vi "__Test_LvDataToMemory_PTR.vi"() -> ()   [LabVIEW 2019]
uses:
  Private/LvDataToMemory_PTR.vi
  __cvi/__TEST_CVI_Prj_PTR/TEST_DataType.dll
  Memory Data Access.lvlib
panel:
  out "Ret_Cluster":i32
  out "Ret_ArrayWav":u32
  out "Ret_Waveform":u32
  out "Ret_TimeStamp":dbl
  out "Ret_ArrayStr":u32
  out "ByteArray":u8[](array[numeric])
  out "Ret_ArrayDBL":u32
  out "Ret_Path":i32
  out "Ret_Str":i32
  out "Ret_Boolean":u8
  out "Ret_DBL":dbl
  out "Ret_I32":i32
  out "Ret_U32":u32
  in  "Enum":T1(ring)
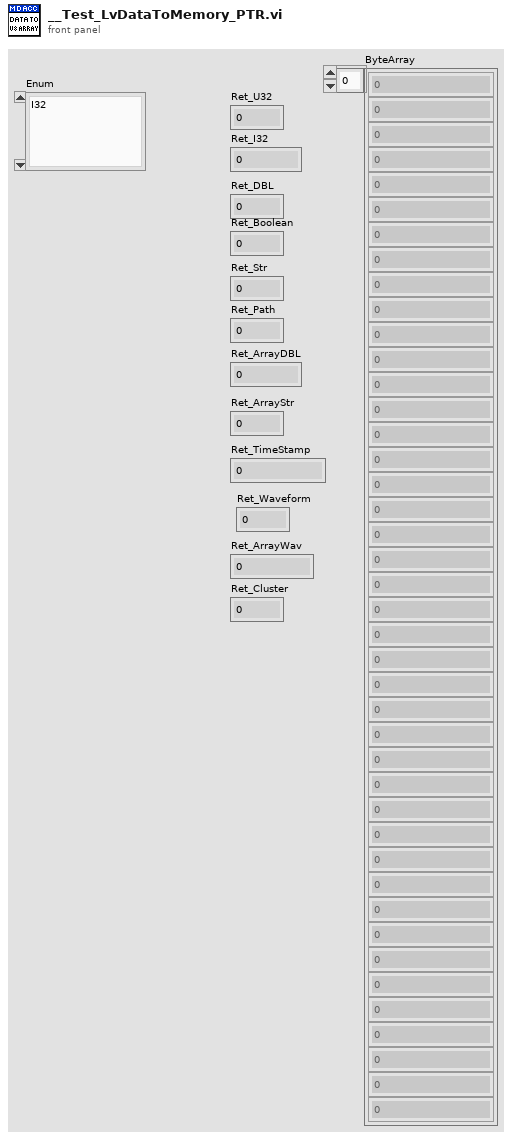
[diagram p1: front panel]
types:
  T1 = enum16{"I32", "U32", "DBL", "String", "Cluster", "Array_Str", "Array_DBL", "Array_Waveform", "Bool", "TimeStamp", "Waveform", "Path"}
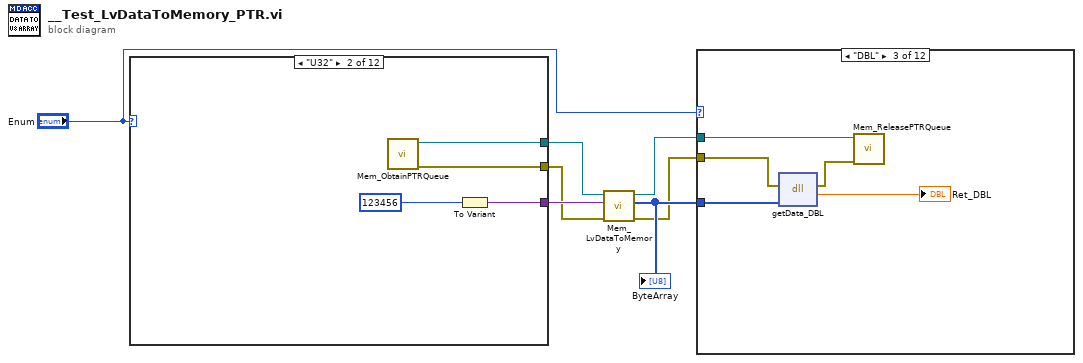
[diagram p0: block diagram]
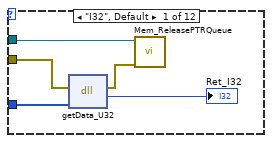
[diagram p2: hidden frame]
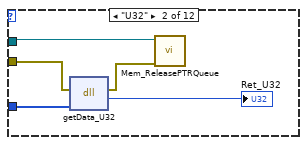
[diagram p3: hidden frame]
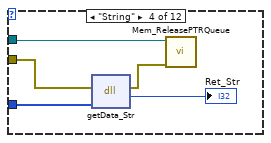
[diagram p4: hidden frame]
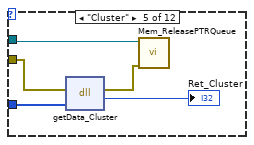
[diagram p5: hidden frame]
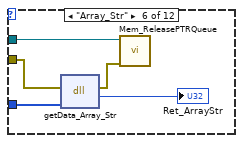
[diagram p6: hidden frame]
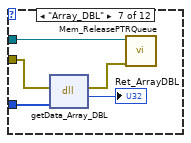
[diagram p7: hidden frame]
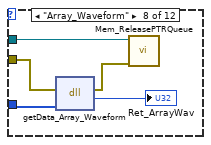
[diagram p8: hidden frame]
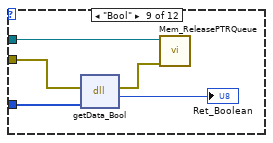
[diagram p9: hidden frame]
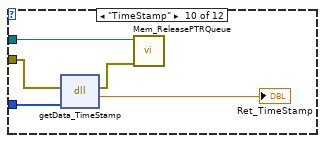
[diagram p10: hidden frame]
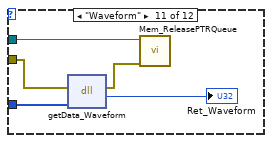
[diagram p11: hidden frame]
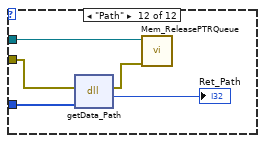
[diagram p12: hidden frame]
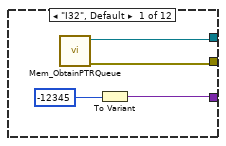
[diagram p13: hidden frame]
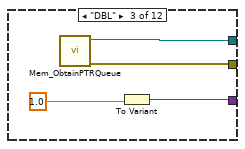
[diagram p14: hidden frame]
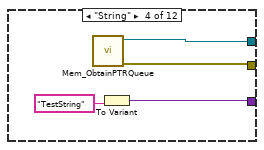
[diagram p15: hidden frame]
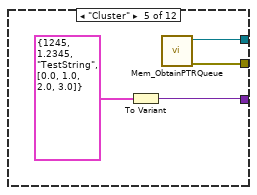
[diagram p16: hidden frame]
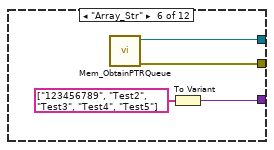
[diagram p17: hidden frame]
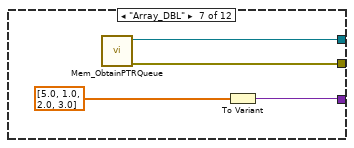
[diagram p18: hidden frame]
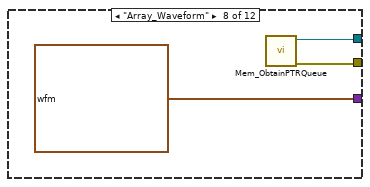
[diagram p19: hidden frame]
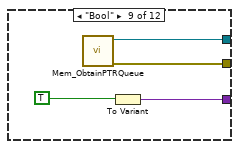
[diagram p20: hidden frame]
diagram:
  n1 = case shown="\"U32\"" "Enum" {
    tunnel: [w11 w15 w19 w23 w27 w30 w35 waveform(dbl)[] [{"t0"=timestamp(3705278400 s since 1904-01-01), "dt"=1.0, "Y"=[1.0, 2.0, 3.0]}, {"t0"=timestamp(3705278400 s since 1904-01-01), "dt"=1.0, "Y"=[4.0, 5.0, 6.0, 7.0]}] w42 w46 w50 w54] -> w7
    tunnel: [w9 w13 w17 w21 w25 w29 w33 w37 w40 w44 w48 w52] -> w3
    tunnel: [w8 w12 w16 w20 w24 w28 w32 w36 w39 w43 w47 w51] -> w2
    frame "I32", Default {
      n2 = call "Mem_ObtainPTRQueue.vi"() -> ("error out"=w8:errorcluster, "queue out"=w9:refnum<queue>)  [unwired: 10 in]
      n3 = To Variant(anything=-12345) -> (Variant=w11:variant)
    }
    frame "U32" {
      n4 = call "Mem_ObtainPTRQueue.vi"() -> ("error out"=w12:errorcluster, "queue out"=w13:refnum<queue>)  [unwired: 10 in]
      n5 = To Variant(anything=u32 123456) -> (Variant=w15:variant)
    }
    frame "DBL" {
      n6 = call "Mem_ObtainPTRQueue.vi"() -> ("error out"=w16:errorcluster, "queue out"=w17:refnum<queue>)  [unwired: 10 in]
      n7 = To Variant(anything=1.0) -> (Variant=w19:variant)
    }
    frame "String" {
      n8 = call "Mem_ObtainPTRQueue.vi"() -> ("error out"=w20:errorcluster, "queue out"=w21:refnum<queue>)  [unwired: 10 in]
      n9 = To Variant(anything="TestString") -> (Variant=w23:variant)
    }
    frame "Cluster" {
      n10 = To Variant(anything=cluster{i32, dbl, string, dbl[]} {1245, 1.2345, "TestString", [0.0, 1.0, 2.0, 3.0]}) -> (Variant=w27:variant)
      n11 = call "Mem_ObtainPTRQueue.vi"() -> ("error out"=w24:errorcluster, "queue out"=w25:refnum<queue>)  [unwired: 10 in]
    }
    frame "Array_Str" {
      n12 = call "Mem_ObtainPTRQueue.vi"() -> ("error out"=w28:errorcluster, "queue out"=w29:refnum<queue>)  [unwired: 10 in]
      n13 = To Variant(anything=string[] ["123456789", "Test2", "Test3", "Test4", "Test5"]) -> (Variant=w30:variant)
    }
    frame "Array_DBL" {
      n14 = call "Mem_ObtainPTRQueue.vi"() -> ("error out"=w32:errorcluster, "queue out"=w33:refnum<queue>)  [unwired: 10 in]
      n15 = To Variant(anything=dbl[] [5.0, 1.0, 2.0, 3.0]) -> (Variant=w35:variant)
    }
    frame "Array_Waveform" {
      n16 = call "Mem_ObtainPTRQueue.vi"() -> ("error out"=w36:errorcluster, "queue out"=w37:refnum<queue>)  [unwired: 10 in]
    }
    frame "Bool" {
      n17 = call "Mem_ObtainPTRQueue.vi"() -> ("error out"=w39:errorcluster, "queue out"=w40:refnum<queue>)  [unwired: 10 in]
      n18 = To Variant(anything=TRUE) -> (Variant=w42:variant)
    }
    frame "TimeStamp" {
      n19 = call "Mem_ObtainPTRQueue.vi"() -> ("error out"=w43:errorcluster, "queue out"=w44:refnum<queue>)  [unwired: 10 in]
      n20 = To Variant(anything=timestamp(3438133200 s since 1904-01-01)) -> (Variant=w46:variant)
    }
    frame "Waveform" {
      n21 = call "Mem_ObtainPTRQueue.vi"() -> ("error out"=w47:errorcluster, "queue out"=w48:refnum<queue>)  [unwired: 10 in]
      n22 = To Variant(anything=waveform(dbl) {"t0"=timestamp(3722126400 s since 1904-01-01), "dt"=1.0, "Y"=[1.0, 2.0, 3.0, 4.0]} ("Waveform")) -> (Variant=w50:variant)
    }
    frame "Path" {
      n23 = call "Mem_ObtainPTRQueue.vi"() -> ("error out"=w51:errorcluster, "queue out"=w52:refnum<queue>)  [unwired: 10 in]
      n24 = To Variant(anything=path "C:/Test/File") -> (Variant=w54:variant)
    }
  }
  n25 = call-poly "Mem_LvDataToMemory.vi"("error in (no error)"=w2, "Payload"=w7, "AddrQueueIn"=w3) -> ("error out"=w4:errorcluster, "ByteArray"=w5:u8[], "AddrQueueOut"=w1:refnum<queue>)  [unwired: 5 in, 1 out]
  "ByteArray" <- w5
  n26 = case shown="\"DBL\"" "Enum" {
    tunnel: w5 -> [w59 w64 w69 w74 w79 w84 w89 w94 w99 w104 w109 w114]
    tunnel: w1 -> [w56 w61 w66 w71 w76 w80 w86 w90 w96 w101 w106 w111]
    tunnel: w4 -> [w57 w62 w67 w72 w77 w82 w87 w92 w97 w102 w107 w112]
    frame "I32", Default {
      n27 = dll-call lib="D:/Workspace/_TEST/Memory-Data-Access/__cvi/__TEST_CVI_Prj_PTR/TEST_DataType.dll" fn="getData_U32"(error in=w57, "Para"=w59) -> (error out=w55:errorcluster, "return type"=→"Ret_I32":i32)  [unwired: 3 in, 1 out]
      n28 = call "Mem_ReleasePTRQueue.vi"("error in (no error)"=w55, "AddrQueueIn"=w56) -> ()  [unwired: 9 in, 1 out]
    }
    frame "U32" {
      n29 = dll-call lib="D:/Workspace/_TEST/Memory-Data-Access/__cvi/__TEST_CVI_Prj_PTR/TEST_DataType.dll" fn="getData_U32"(error in=w62, "Para"=w64) -> (error out=w60:errorcluster, "return type"=→"Ret_U32":u32)  [unwired: 3 in, 1 out]
      n30 = call "Mem_ReleasePTRQueue.vi"("error in (no error)"=w60, "AddrQueueIn"=w61) -> ()  [unwired: 9 in, 1 out]
    }
    frame "DBL" {
      n31 = dll-call lib="D:/Workspace/_TEST/Memory-Data-Access/__cvi/__TEST_CVI_Prj_PTR/TEST_DataType.dll" fn="getData_DBL"(error in=w67, "Para"=w69) -> (error out=w65:errorcluster, "return type"=→"Ret_DBL":dbl)  [unwired: 3 in, 1 out]
      n32 = call "Mem_ReleasePTRQueue.vi"("error in (no error)"=w65, "AddrQueueIn"=w66) -> ()  [unwired: 9 in, 1 out]
    }
    frame "String" {
      n33 = dll-call lib="D:/Workspace/_TEST/Memory-Data-Access/__cvi/__TEST_CVI_Prj_PTR/TEST_DataType.dll" fn="getData_Str"(error in=w72, "Para"=w74) -> (error out=w70:errorcluster, "return type"=→"Ret_Str":i32)  [unwired: 3 in, 1 out]
      n34 = call "Mem_ReleasePTRQueue.vi"("error in (no error)"=w70, "AddrQueueIn"=w71) -> ()  [unwired: 9 in, 1 out]
    }
    frame "Cluster" {
      n35 = dll-call lib="D:/Workspace/_TEST/Memory-Data-Access/__cvi/__TEST_CVI_Prj_PTR/TEST_DataType.dll" fn="getData_Cluster"(error in=w77, "Para"=w79) -> (error out=w75:errorcluster, "return type"=→"Ret_Cluster":i32)  [unwired: 3 in, 1 out]
      n36 = call "Mem_ReleasePTRQueue.vi"("error in (no error)"=w75, "AddrQueueIn"=w76) -> ()  [unwired: 9 in, 1 out]
    }
    frame "Array_Str" {
      n37 = dll-call lib="D:/Workspace/_TEST/Memory-Data-Access/__cvi/__TEST_CVI_Prj_PTR/TEST_DataType.dll" fn="getData_Array_Str"(error in=w82, "Para"=w84) -> (error out=w81:errorcluster, "return type"=→"Ret_ArrayStr":u32)  [unwired: 3 in, 1 out]
      n38 = call "Mem_ReleasePTRQueue.vi"("error in (no error)"=w81, "AddrQueueIn"=w80) -> ()  [unwired: 9 in, 1 out]
    }
    frame "Array_DBL" {
      n39 = dll-call lib="D:/Workspace/_TEST/Memory-Data-Access/__cvi/__TEST_CVI_Prj_PTR/TEST_DataType.dll" fn="getData_Array_DBL"(error in=w87, "Para"=w89) -> (error out=w85:errorcluster, "return type"=→"Ret_ArrayDBL":u32)  [unwired: 3 in, 1 out]
      n40 = call "Mem_ReleasePTRQueue.vi"("error in (no error)"=w85, "AddrQueueIn"=w86) -> ()  [unwired: 9 in, 1 out]
    }
    frame "Array_Waveform" {
      n41 = dll-call lib="D:/Workspace/_TEST/Memory-Data-Access/__cvi/__TEST_CVI_Prj_PTR/TEST_DataType.dll" fn="getData_Array_Waveform"(error in=w92, "Para"=w94) -> (error out=w91:errorcluster, "return type"=→"Ret_ArrayWav":u32)  [unwired: 3 in, 1 out]
      n42 = call "Mem_ReleasePTRQueue.vi"("error in (no error)"=w91, "AddrQueueIn"=w90) -> ()  [unwired: 9 in, 1 out]
    }
    frame "Bool" {
      n43 = dll-call lib="D:/Workspace/_TEST/Memory-Data-Access/__cvi/__TEST_CVI_Prj_PTR/TEST_DataType.dll" fn="getData_Bool"(error in=w97, "Para"=w99) -> (error out=w95:errorcluster, "return type"=→"Ret_Boolean":u8)  [unwired: 3 in, 1 out]
      n44 = call "Mem_ReleasePTRQueue.vi"("error in (no error)"=w95, "AddrQueueIn"=w96) -> ()  [unwired: 9 in, 1 out]
    }
    frame "TimeStamp" {
      n45 = dll-call lib="D:/Workspace/_TEST/Memory-Data-Access/__cvi/__TEST_CVI_Prj_PTR/TEST_DataType.dll" fn="getData_TimeStamp"(error in=w102, "Para"=w104) -> (error out=w100:errorcluster, "return type"=→"Ret_TimeStamp":dbl)  [unwired: 3 in, 1 out]
      n46 = call "Mem_ReleasePTRQueue.vi"("error in (no error)"=w100, "AddrQueueIn"=w101) -> ()  [unwired: 9 in, 1 out]
    }
    frame "Waveform" {
      n47 = dll-call lib="D:/Workspace/_TEST/Memory-Data-Access/__cvi/__TEST_CVI_Prj_PTR/TEST_DataType.dll" fn="getData_Waveform"(error in=w107, "Para"=w109) -> (error out=w105:errorcluster, "return type"=→"Ret_Waveform":u32)  [unwired: 3 in, 1 out]
      n48 = call "Mem_ReleasePTRQueue.vi"("error in (no error)"=w105, "AddrQueueIn"=w106) -> ()  [unwired: 9 in, 1 out]
    }
    frame "Path" {
      n49 = dll-call lib="D:/Workspace/_TEST/Memory-Data-Access/__cvi/__TEST_CVI_Prj_PTR/TEST_DataType.dll" fn="getData_Path"(error in=w112, "Para"=w114) -> (error out=w110:errorcluster, "return type"=→"Ret_Path":i32)  [unwired: 3 in, 1 out]
      n50 = call "Mem_ReleasePTRQueue.vi"("error in (no error)"=w110, "AddrQueueIn"=w111) -> ()  [unwired: 9 in, 1 out]
    }
  }
